vi "Test Random Flag will repeat or not.vi"() -> ()   [LabVIEW 2020]
panel:
  out "time(s)":dbl
  out "*(type *) &x":string
  out "Numeric":i32
  out "number: 0 to 1":u64 format="%.0x"
  out "number (0 to 1)":u64 format="%.0x"
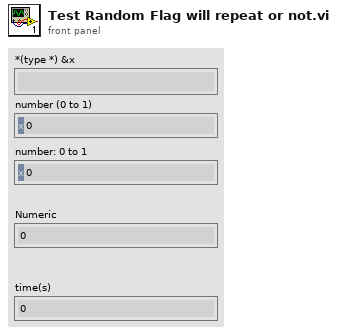
[diagram p1: front panel]
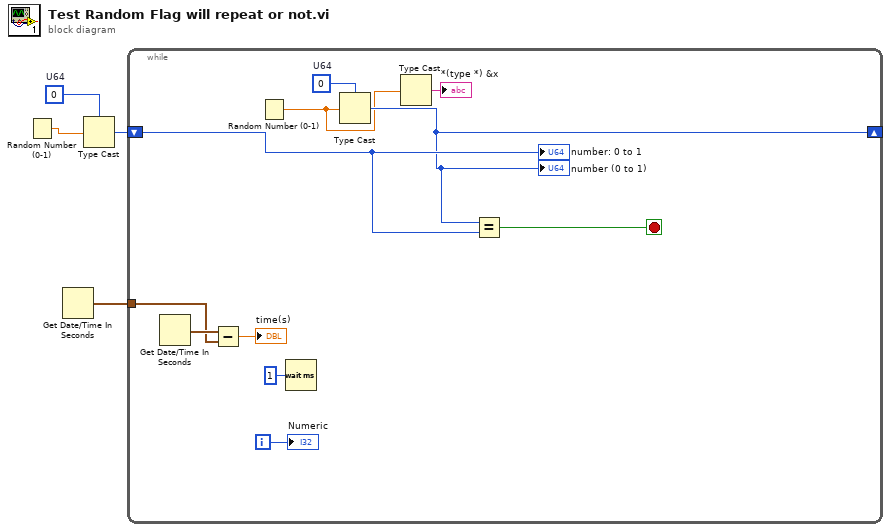
[diagram p0: block diagram]
diagram:
  w2 = u64 0  # U64
  n1 = Random Number (0-1)() -> (number: 0 to 1=w4:dbl)
  n2 = Get Date/Time In Seconds() -> (seconds since 1Jan1904=w1:timestamp)
  n3 = Type Cast(type=w2, x=w4) -> (*(type *) &x=w3:u64)
  n4 = while {
    shift-right: [w11] -> _
    shift-left: w3 -> [w15]
    tunnel: w1 -> [w6]
    i -> [w13]
    stop <- w14 stop-if-true
    w10 = u64 0  # U64
    n5 = Get Date/Time In Seconds() -> (seconds since 1Jan1904=w7:timestamp)
    n6 = Subtract(x=w7, y=w6) -> (x-y=→"time(s)":dbl)
    n7 = Random Number (0-1)() -> (number: 0 to 1=w9:dbl)
    n8 = Wait (ms)(milliseconds to wait=u32 1) -> ()  [unwired: 1 out]
    n9 = Type Cast(type=w10, x=w9) -> (*(type *) &x=w11:u64)
    "number (0 to 1)" <- w11
    n10 = Type Cast(x=w9) -> (*(type *) &x=→"*(type *) &x":string)  [unwired: 1 in]
    n11 = Equal?(x=w11, y=w15) -> (x = y?=w14:bool)
    "number: 0 to 1" <- w15
    "Numeric" <- w13
  }
